vi "Begin.vi"(8 "error in":errorcluster) -> (0 "error out":errorcluster)   [LabVIEW 2019]
doc: "Called before other user functions, this VI is expected to open initial I/O refnums, load in file data, and do all program initialization. Notice that the <B>error out</B> terminal is simply used for data flow. Wiring it to other structures or subVIs ensures that this VI runs first."
uses:
  <vilib>/Rock Robotics/WPI/DriverStation/WPI_DriverStationRobotMode2.ctl
  Robot Global Data.vi
  <vilib>/Rock Robotics/Network Tables/NT Write String Array.vi
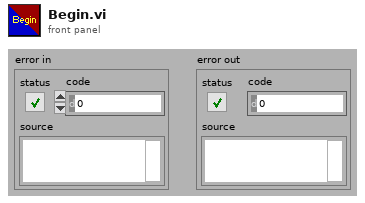
[diagram p1: front panel]
types:
  T1 = typedef "WPI_DriverStationRobotMode2.ctl" = enum16{"Autonomous Disabled", "Autonomous Enabled", "Teleop Disabled", "Teleop Enabled", "Disconnected", "Finish", "Test Disabled", "Test Enabled", "Emergency Stopped"}
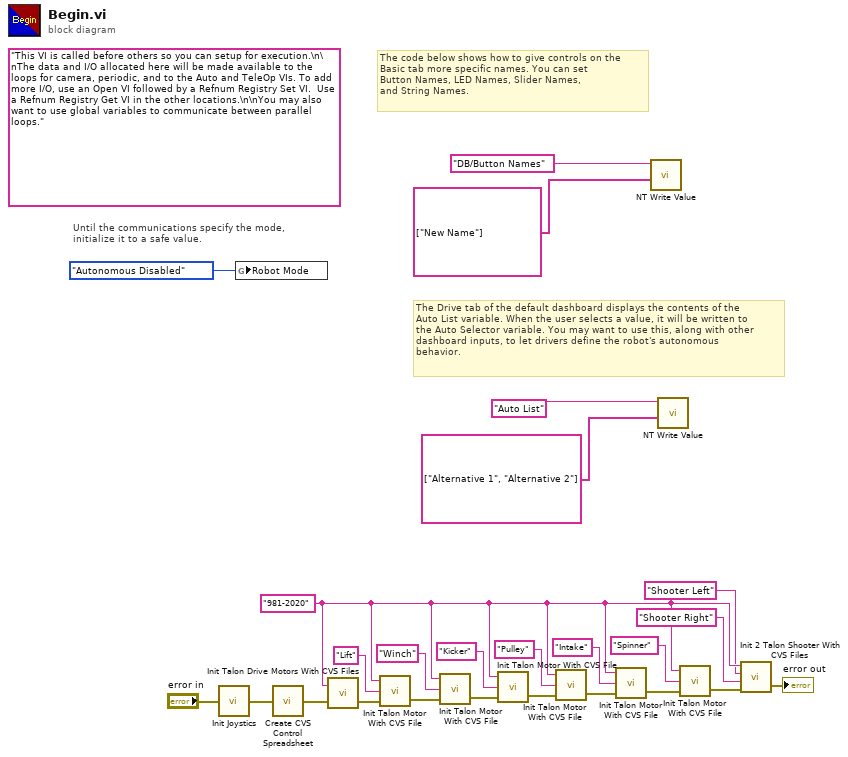
[diagram p0: block diagram]
diagram:
  w3 = "981-2020" ("Robot ID")
  (unwired) "This VI is called before others so you can setup for execution.\n\nThe data and I/O allocated here will be made available to the loops for camera, periodic, and to the Auto and TeleOp VIs. To add more I/O, use an Open VI followed by a Refnum Registry Set VI.  Use a Refnum Registry Get VI in the other locations.\n\nYou may also want to use global variables to communicate between parallel loops."
  # "The Drive tab of the default dashboard displays the contents of the\nAuto List variable. When the user selects a value, it will be written to\nthe Auto Selector variable. You may want to use this, along with other\ndashboard inputs, to let drivers define the robot's autonomous\nbehavior."
  # "The code below shows how to give controls on the\nBasic tab more specific names. You can set\nButton Names, LED Names, Slider Names,\nand String Names."
  # "Until the communications specify the mode,\ninitialize it to a safe value."
  n1 = call "Init Joystics.vi"("error in"="error in") -> ("error out"=w20:errorcluster)
  n2 = global write "Robot Global Data.vi" "Robot Mode"(WPI_DriverStationRobotMode2."Autonomous Disabled" ("Robot Mode")) -> ()
  n3 = call "Create CVS Control Spreadsheet.vi"("error in"=w20) -> ("error out"=w19:errorcluster)
  n4 = call "Init Talon Drive Motors With CVS Files.vi"("error in"=w19, "Robot ID"=w3) -> ("error out"=w14:errorcluster)  [unwired: 1 out]
  n5 = call "Init Talon Motor With CVS File.vi"("error in"=w14, "Motor ID"="Lift", "Robot ID"=w3) -> ("error out"=w15:errorcluster)  [unwired: 1 out]
  n6 = call "Init Talon Motor With CVS File.vi"("error in"=w15, "Motor ID"="Winch", "Robot ID"=w3) -> ("error out"=w12:errorcluster)  [unwired: 1 out]
  n7 = call "Init Talon Motor With CVS File.vi"("error in"=w12, "Motor ID"="Kicker", "Robot ID"=w3) -> ("error out"=w11:errorcluster)  [unwired: 1 out]
  n8 = call "Init Talon Motor With CVS File.vi"("error in"=w11, "Motor ID"="Pulley", "Robot ID"=w3) -> ("error out"=w7:errorcluster)  [unwired: 1 out]
  n9 = call "Init Talon Motor With CVS File.vi"("error in"=w7, "Motor ID"="Intake", "Robot ID"=w3) -> ("error out"=w6:errorcluster)  [unwired: 1 out]
  n10 = call-poly <vilib>:"NT Write Value.vi"("String Array"=string[] ["New Name"], "Name"="DB/Button Names") -> ()  [unwired: 9 in, 1 out]
  n11 = call-poly <vilib>:"NT Write Value.vi"("String Array"=string[] ["Alternative 1", "Alternative 2"], "Name"="Auto List") -> ()  [unwired: 9 in, 1 out]
  n12 = call "Init Talon Motor With CVS File.vi"("error in"=w6, "Motor ID"="Spinner", "Robot ID"=w3) -> ("error out"=w5:errorcluster)  [unwired: 1 out]
  n13 = call "Init 2 Talon Shooter With CVS Files.vi"("error in"=w5, "Shooter Right ID"="Shooter Right", "Shooter Left ID"="Shooter Left", "Robot ID"=w3) -> ("error out"=→"error out":errorcluster)  [unwired: 1 out]
